vi "Get Raw Data Folder.vi"(1 "Raw data file":path) -> (0 "Main Raw Data Folder":path)   [LabVIEW 2020]
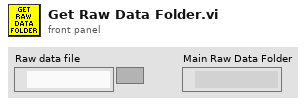
[diagram p1: front panel]
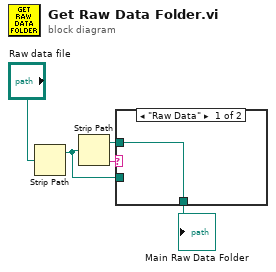
[diagram p0: block diagram]
diagram:
  n1 = Strip Path(path="Raw data file") -> (stripped path=w2:path)  [unwired: 1 out]
  n2 = Strip Path(path=w2) -> (stripped path=w5:path, name=w3:string)
  n3 = case shown="\"Raw Data\"" w3 {
    tunnel: w2 -> [_ w7]
    tunnel: [w6 w7] -> w4
    tunnel: w5 -> [w6 _]
    frame "Raw Data" {
    }
    frame Default {
    }
  }
  "Main Raw Data Folder" <- w4
